vi "Frame.CheckErrors.vi"(7 "Existing PIDs":string[](array[string]), 8 "error in (no error)":errorcluster, 9 "ID":u16, 10 "Name":string, 11 "Signals":T1[](array[typedef]) {"Byte Order" items=["Little Endian", "Big Endian"]; "Data Type" items=["Signed", "Unsigned", "IEEE Float"]}) -> (0 "error out":errorcluster, 2 "Error Type":string, 3 "Error?":bool)   [LabVIEW 2024, in "Diagnostics Addon System Explorer.lvlib"]
uses:
  Diagnostics Addon System Explorer.lvlib
  Addon Shared/Types/Signal.ctl
  Addon Shared/Types/XNET.Frame.ctl
  Addon Shared/SubVIs/Constants.vi
  <vilib>/xnet/xnet.llb/XNET Database Create (Cluster).vi
  <vilib>/xnet/xnet.llb/XNET Database Delete (Cluster).vi
  <vilib>/xnet/xnet.llb/XNET Database Close (Database).vi
  Addon Shared/Diagnostics Addon Shared.lvlib
  <resource>/objmgr/xnet.rc
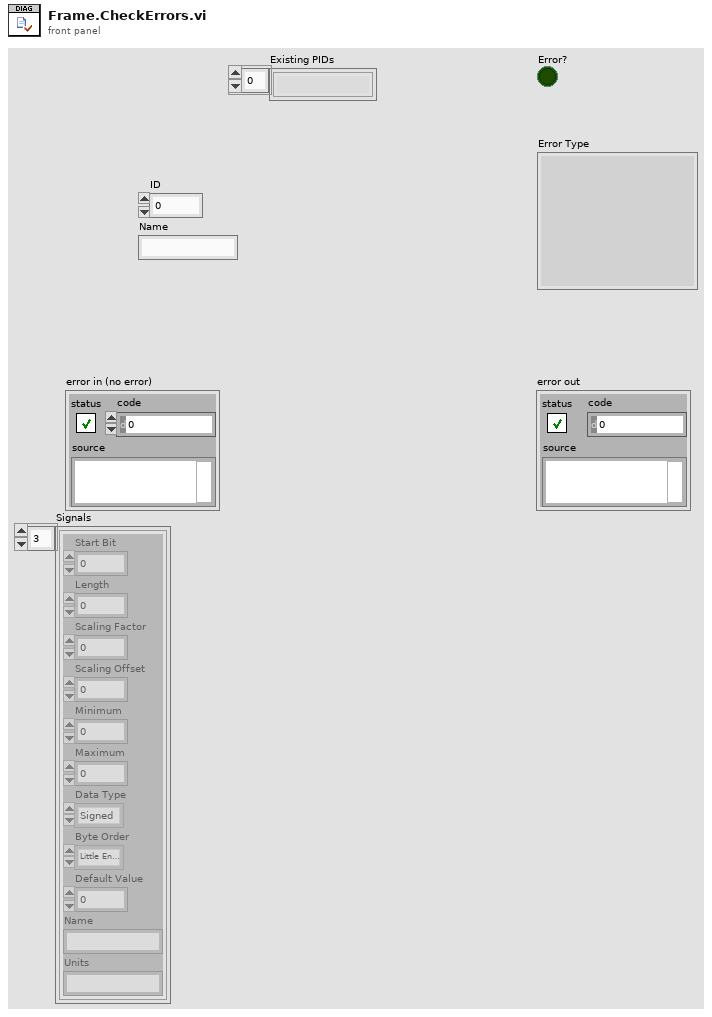
[diagram p1: front panel]
types:
  T1 = typedef "Diagnostics Addon Shared.lvlib/Signal.ctl" = cluster{"Start Bit":u32, "Length":u32, "Scaling Factor":dbl, "Scaling Offset":dbl, "Minimum":dbl, "Maximum":dbl, "Data Type":u32, "Byte Order":u32, "Default Value":dbl, "Name":string, "Units":string}
  T2 = enum16{"CheckSignalNames", "CheckBits", "CheckName"}[]
  T3 = typedef "Diagnostics Addon Shared.lvlib/XNET.Frame.ctl" = cluster{"Frame name":string, "Identifier":u32, "Payload Length":u32, "Timing Type":u32, "Transmit Time":dbl, "Extended Identifier?":bool, "Comment":string, "IO Mode":u32}
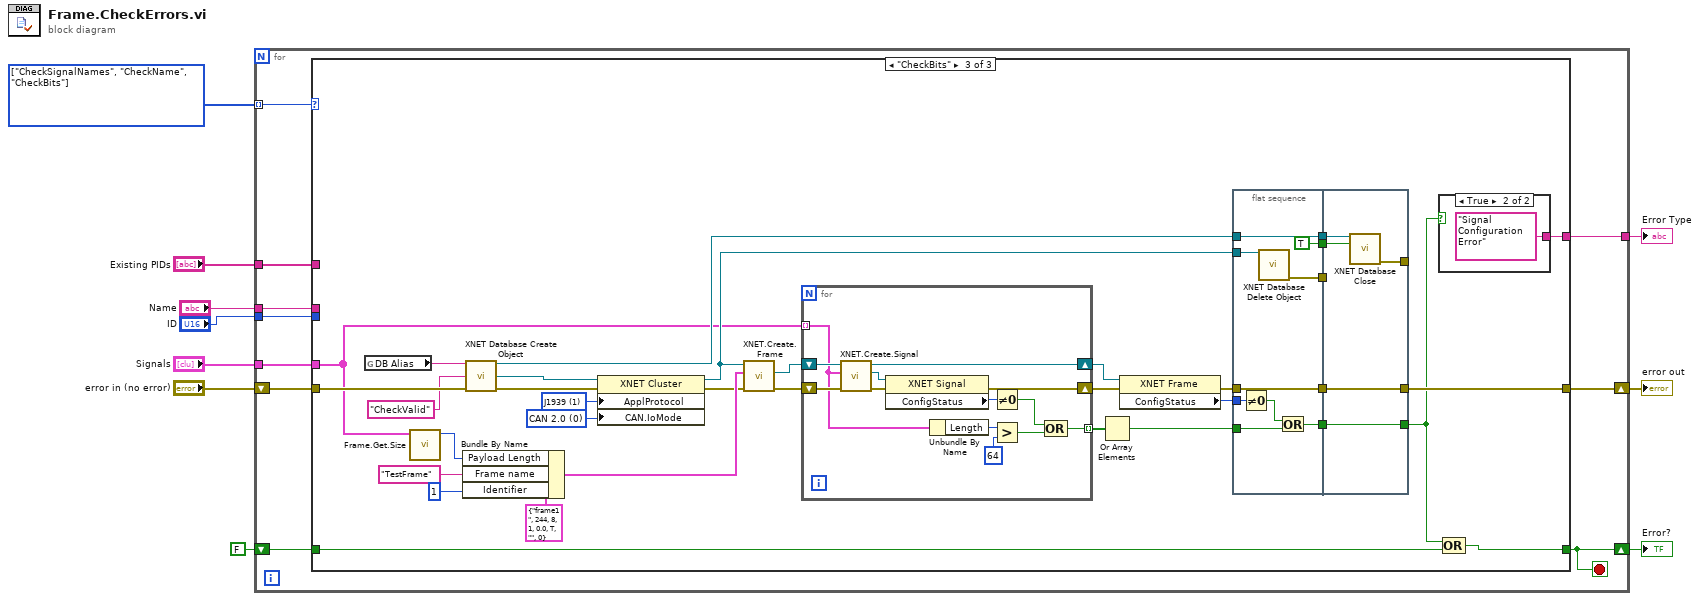
[diagram p0: block diagram]
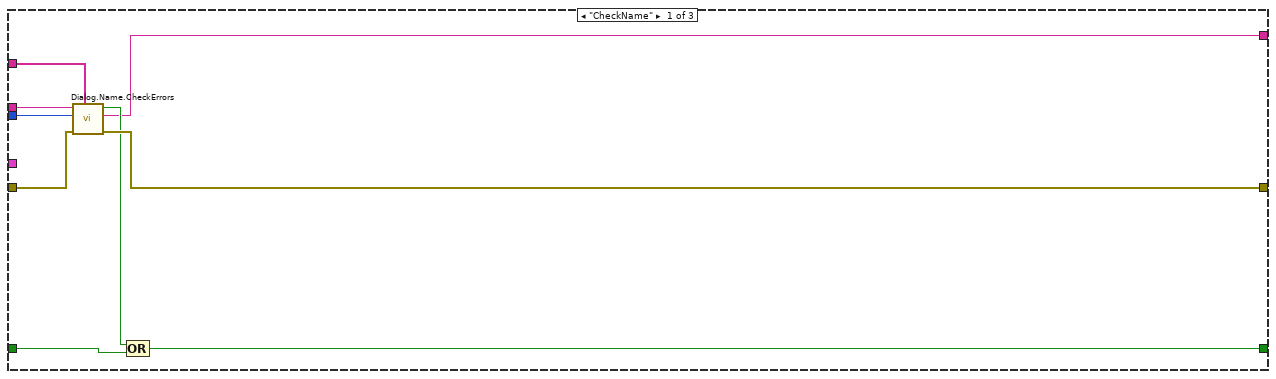
[diagram p2: hidden frame]
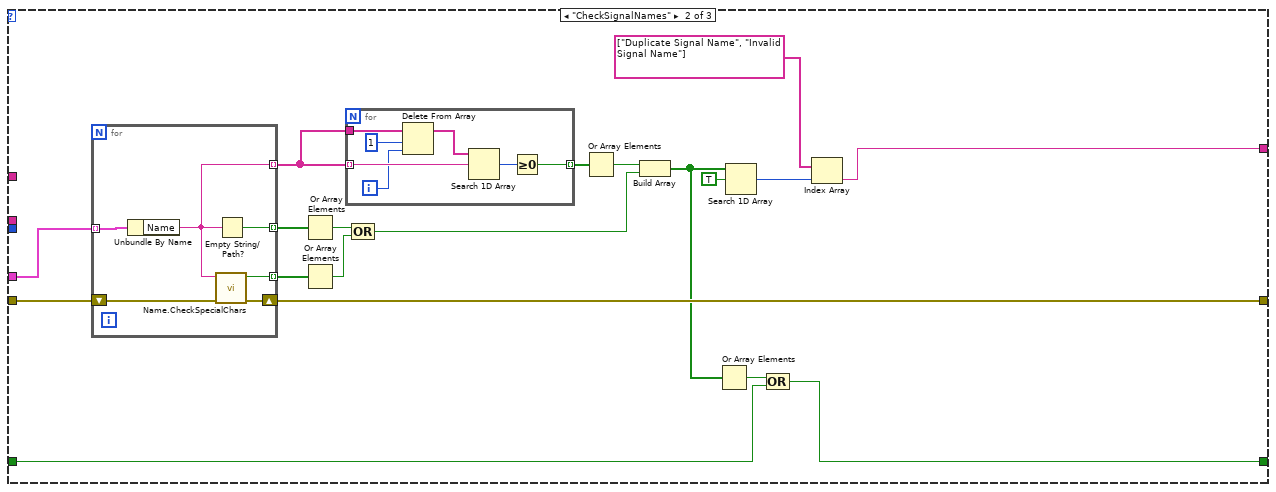
[diagram p3: hidden frame]
diagram:
  w10 = T2 [enum."CheckSignalNames", enum."CheckName", enum."CheckBits"] items=["CheckSignalNames", "CheckBits", "CheckName"]
  n1 = for {
    tunnel: w10 -> [w20] mode=indexing
    shift-right: [w17] -> w7
    shift-left: "error in (no error)" -> [w16]
    tunnel: "Signals" -> [w19]
    shift-right: [w11] -> w8
    shift-left: FALSE -> [w18]
    tunnel: "Existing PIDs" -> [w15]
    tunnel: "Name" -> [w14]
    tunnel: "ID" -> [w13]
    tunnel: [w12] -> w5
    stop <- w11 stop-if-true
    n2 = case shown="\"CheckBits\"" w20 {
      tunnel: w19 -> [_ w48 w63]
      tunnel: [w26 w37 w95] -> w11
      tunnel: w18 -> [w27 w36 w62]
      tunnel: [w28 w41 w94] -> w17
      tunnel: w16 -> [w29 w42 w91]
      tunnel: w15 -> [w23 _ _]
      tunnel: w14 -> [w21 _ _]
      tunnel: w13 -> [w22 _ _]
      tunnel: [w24 w30 w93] -> w12
      frame "CheckName" {
        n3 = call "Dialog.Name.CheckErrors.vi"("Existing Frames"=w23, "error in (no error)"=w29, "ID"=w22, "Name"=w21) -> ("error out"=w28:errorcluster, "Error"=w24:string, "Error?"=w25:bool)  [unwired: 5 in]
        n4 = Compound Arithmetic op=OR(w25, w27) -> (w26:bool)
      }
      frame "CheckSignalNames" {
        n5 = for {
          tunnel: w48 -> [w61] mode=indexing
          tunnel: [w58] -> w47 mode=indexing
          tunnel: [w60] -> w46 mode=indexing
          tunnel: [w59] -> w43 mode=indexing
          shift-right: [w56] -> w41
          shift-left: w42 -> [w57]
          n6 = Unbundle By Name(w61) -> ("Name"=w60:string)
          n7 = call "Name.CheckSpecialChars.vi"("error in"=w57, "Signal Name"=w60) -> ("error out"=w56:errorcluster, "Special Character?"=w59:bool)  [unwired: 8 in]
          n8 = Empty String/Path?(string/path=w60) -> (empty?=w58:bool)
        }
        n9 = Or Array Elements(Boolean array=w47) -> (logical OR=w34:bool)
        n10 = Or Array Elements(Boolean array=w43) -> (logical OR=w35:bool)
        n11 = for {
          tunnel: w46 -> [w50]
          tunnel: w46 -> [w55] mode=indexing
          tunnel: [w53] -> w45 mode=indexing
          i -> [w51]
          n12 = Delete From Array(array=w50, length=1, index=w51) -> (array with subset deleted=w49:string[])  [unwired: 1 out]
          n13 = Search 1D Array(1D array=w49, element=w55) -> (index of element=w54:i32)  [unwired: 1 in]
          n14 = Greater Or Equal To 0?(x=w54) -> (x >= 0?=w53:bool)
        }
        n15 = Compound Arithmetic op=OR(w34, w35) -> (w33:bool)
        n16 = Or Array Elements(Boolean array=w45) -> (logical OR=w44:bool)
        n17 = Build Array(w44, w33) -> (w39:bool[])
        n18 = Or Array Elements(Boolean array=w39) -> (logical OR=w38:bool)
        n19 = Search 1D Array(1D array=w39, element=TRUE) -> (index of element=w32:i32)  [unwired: 1 in]
        n20 = Compound Arithmetic op=OR(w38, w36) -> (w37:bool)
        n21 = Index Array(array=string[] ["Duplicate Signal Name", "Invalid Signal Name"], index=w32) -> (element=w30:string)
      }
      frame "CheckBits" {
        w65 = u32 0 items=["CAN 2.0", "CAN FD", "CAN FD+BRS"] ("CAN:I/O Mode")
        w66 = u32 1 items=["None", "J1939"] ("Application Protocol")
        n22 = global read "Constants.vi" "DB Alias"() -> (w77:string)
        n23 = call "Frame.Get.Size.vi"("Parameters"=w63) -> ("Bytes"=w64:u32)  [unwired: 10 in]
        n24 = Bundle By Name(cluster=T3 {"Frame name"="frame1", "Identifier"=244, "Payload Length"=8, "Timing Type"=1, "Transmit Time"=0.0, "Extended Identifier?"=TRUE, "Comment"="", "IO Mode"=0} ("CAN Frame"), "Payload Length"=w64, "Frame name"="TestFrame" ("cluster name"), "Identifier"=u32 1) -> (w80:T3)
        n25 = call-poly <vilib>:"XNET Database Create Object.vi"("database in"=w77, "cluster name"="CheckValid", "error in (no error)"=w91) -> ("database out"=w74:refnum<k21>, "cluster out"=w75:refnum<k21>, "error out"=w68:errorcluster)  [unwired: 10 in]
        n26 = property class="XNET Cluster"(reference=w75, error in=w68, "ApplProtocol"=w66, "CAN.IoMode"=w65) -> (reference out=w69:refnum<k21>, error out=w67:errorcluster)
        n27 = call "XNET.Create.Frame.vi"("error in"=w67, "CAN Frame"=w80, "cluster in"=w69) -> ("error out"=w83:errorcluster, "frame out"=w84:refnum<k21>)  [unwired: 6 in, 1 out]
        n28 = for {
          tunnel: [w98] -> w72 mode=indexing
          shift-right: [w105] -> w78
          shift-left: w84 -> [w107]
          shift-right: [w108] -> w85
          shift-left: w83 -> [w106]
          tunnel: w63 -> [w100] mode=indexing
          n29 = call "XNET.Create.Signal.vi"("error in"=w106, "Signal"=w100, "frame in"=w107) -> ("error out"=w102:errorcluster, "signal out"=w103:refnum<k21>, "frame out"=w105:refnum<k21>)  [unwired: 6 in]
          n30 = property class="XNET Signal"(reference=w103, error in=w102) -> (error out=w108:errorcluster, "ConfigStatus"=w101:i32)  [unwired: 1 out]
          n31 = Unbundle By Name(w100) -> ("Length"=w99:u32)
          n32 = Not Equal To 0?(x=w101) -> (x != 0?=w104:bool)
          n33 = Greater?(x=w99, y=u32 64) -> (0:w97:bool)
          n34 = Compound Arithmetic op=OR(w104, w97) -> (w98:bool)
        }
        n35 = Or Array Elements(Boolean array=w72) -> (logical OR=w70:bool)
        n36 = property class="XNET Frame"(reference=w78, error in=w85) -> (error out=w71:errorcluster, "ConfigStatus"=w73:i32)  [unwired: 1 out]
        n37 = flat-sequence {
          tunnel: w71 -> [w116]
          tunnel: w69 -> [w117]
          tunnel: w74 -> [w115]
          tunnel: [w116] -> w90
          tunnel: [w115] -> w89
          tunnel: [w114] -> w88
          tunnel: w73 -> [w112]
          tunnel: w70 -> [w109]
          tunnel: [w111] -> w87
          tunnel: [TRUE ("close all? (true)")] -> w86
          tunnel: w90 -> [w122]
          tunnel: w89 -> [w121]
          tunnel: w88 -> [_]
          tunnel: w87 -> [w120]
          tunnel: [w122] -> w94
          tunnel: [w120] -> w92
          tunnel: [w119] -> _
          tunnel: w86 -> [w118]
          frame #0 {
            n38 = Not Equal To 0?(x=w112) -> (x != 0?=w113:bool)
            n39 = call-poly <vilib>:"XNET Database Delete Object.vi"("cluster in"=w117) -> ("error out"=w114:errorcluster)  [unwired: 14 in]
            n40 = Or(x=w113, y=w109) -> (x .or. y?=w111:bool)
          }
          frame #1 {
            n41 = call-poly <vilib>:"XNET Database Close.vi"("database in"=w121, "close all? (true)"=w118) -> ("error out"=w119:errorcluster)  [unwired: 13 in]
          }
        }
        n42 = case shown="True" w92 {
          tunnel: [_ "Signal Configuration Error"] -> w93
          frame False {
          }
          frame True {
          }
        }
        n43 = Compound Arithmetic op=OR(w92, w62) -> (w95:bool)
      }
    }
  }
  "Error?" <- w8
  "error out" <- w7
  "Error Type" <- w5
